vi "Handle Custom Device Name Change.vi"(8 "error in (no error)":errorcluster, 10 "Main Page Controls":T2, 11 "Item Ref in":T1 format="%.0x") -> (0 "error out":errorcluster, 3 "Item Ref out":T1 format="%.0x")   [LabVIEW 2020, in "NI-SWITCH System Explorer.lvlib"]
uses:
  NI-SWITCH System Explorer.lvlib
  Main Page Controls.ctl
  <vilib>/NI VeriStand/Custom Device API/Custom Device Item Ref.ctl
  Scripting/NI-SWITCH Scripting.lvlib
  <vilib>/NI VeriStand/Custom Device API/Custom Device API.lvlib
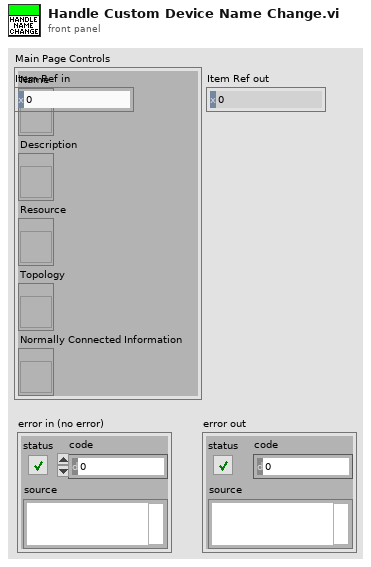
[diagram p1: front panel]
types:
  T1 = typedef "Custom Device API.lvlib/Custom Device Item Ref.ctl" = u64
  T2 = typedef "NI-SWITCH System Explorer.lvlib/Main Page Controls.ctl" = cluster{"Name":refnum<vi>, "Description":refnum<vi>, "Resource":refnum<vi>, "Topology":refnum<vi>, "Normally Connected Information":refnum<vi>}
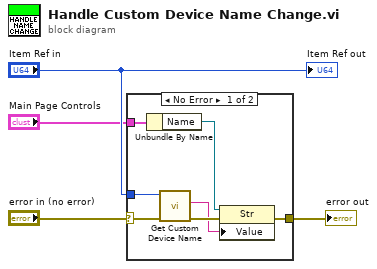
[diagram p0: block diagram]
diagram:
  n1 = case shown="No Error" "error in (no error)" {
    selector: "error in (no error)" -> [w9 w12]
    tunnel: "Item Ref in" -> [w11 _]
    tunnel: [w7 w12] -> w4
    tunnel: "Main Page Controls" -> [w8 _]
    frame No Error {
      n2 = Unbundle By Name(w8) -> ("Name"=w6:refnum<vi>)
      n3 = call "Get Custom Device Name.vi"("error in"=w9, "ni-switch custom device in"=w11) -> ("error out"=w10:errorcluster, "name"=w5:string)  [unwired: 7 in, 1 out]
      n4 = property class="Str"(reference=w6, error in=w10, "Value"=w5) -> (error out=w7:errorcluster)  [unwired: 1 out]
    }
    frame Error {
    }
  }
  "error out" <- w4
  "Item Ref out" <- "Item Ref in"
